vi "close visualizer.vi"(8 "error in (no error)":errorcluster, 10 "Queue in":refnum<queue>, 11 "reference":refnum<vi>) -> (0 "error out":errorcluster)   [LabVIEW 2016, in "FPGA RM System Definition API.lvlib"]
uses:
  FPGA-Resource-Manager-APIs/Source/System Definition/FPGA RM System Definition API.lvlib
  viz_command.ctl
  viz_state.ctl
  visualizer globals.vi
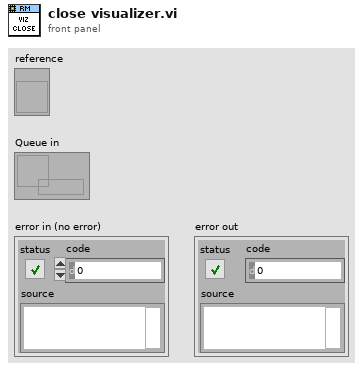
[diagram p1: front panel]
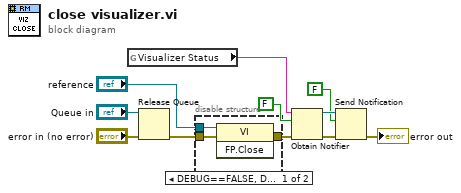
[diagram p0: block diagram]
diagram:
  n1 = global read "visualizer globals.vi" "Visualizer Status"() -> (w7:string)
  n2 = Release Queue(queue="Queue in", error in (no error)="error in (no error)") -> (error out=w11:errorcluster)  [unwired: 1 in, 2 out]
  n3 = disable-structure shown="DEBUG==FALSE, Default" {
    disable-tunnel: w11 -> [w14 w15]
    disable-tunnel: "reference" -> [w13 _]
    disable-tunnel: [w12 w15] -> w2
    frame condition #0 (active) {
      n4 = invoke class="VI" method="FP.Close"(reference=w13, error in=w14) -> (error out=w12:errorcluster)  [unwired: 1 in, 2 out]
    }
    frame condition #1 {
    }
  }
  n5 = Obtain Notifier(name (unnamed)=w7, notification data type=FALSE, error in (no error)=w2) -> (notifier out=w5:refnum<notifier>, error out=w3:errorcluster)  [unwired: 1 in, 1 out]
  n6 = Send Notification(notification=FALSE, notifier=w5, error in (no error)=w3) -> (error out=→"error out":errorcluster)  [unwired: 1 out]
